vi "getModbusSubnetB.vi"(11 "ILCCommunications in":refnum<class "ILCCommunications.lvclass">) -> (2 "ModbusSubnetB":refnum<class "IModbus.lvclass">, 3 "ILCCommunications out":refnum<class "ILCCommunications.lvclass">)   [LabVIEW 2016, in "ILCCommunications.lvclass"]
uses:
  ILCCommunications.lvclass
  Common_RT_Modbus/IModbus/IModbus.lvclass
  ILCCommunications.lvclass/ILCCommunications.ctl
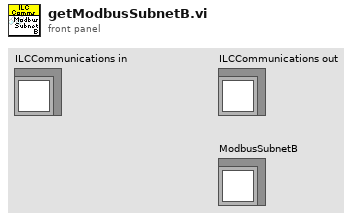
[diagram p1: front panel]
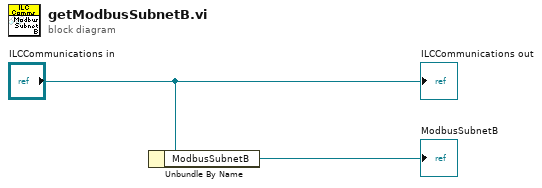
[diagram p0: block diagram]
diagram:
  n1 = Unbundle By Name("ILCCommunications in") -> ("ModbusSubnetB"=→"ModbusSubnetB":refnum<class "IModbus.lvclass">)
  "ILCCommunications out" <- "ILCCommunications in"
